vi "VotingClassifier.vi"(8 "error in":errorcluster) -> (0 "error out":errorcluster, 3 "out":refnum<class "VotingClassifier.lvclass">)   [LabVIEW 2020]
doc: "Soft Voting/Majority Rule classifier for unfitted estimators.\n\n Read more in the :ref:`User Guide <voting_classifier>`.\n\n .. versionadded:: 0.17\n\n Parameters\n ----------\n estimators : list of (str, estimator) tuples\n Invoking the ``fit`` method on the ``VotingClassifier`` will fit clones\n of those original estimators that will be stored in the class attribute\n ``self.estimators_``. An estimator can be set to ``'drop'``\n using ``set_params``.\n\n .. versionchanged:: 0.21\n ``'drop'`` is accepted. Using None was deprecated in 0.22 and\n support was removed in 0.24.\n\n voting : {'hard', 'soft'}, default='hard'\n If 'hard', uses predicted class labels for majority rule voting.\n Else if 'soft', predicts the class label based on the argmax of\n the sums of the predicted probabilities, which is recommended for\n an ensemble of well-calibrated classifiers.\n\n weights : array-like of shape (n_classifiers,), default=None\n Sequence of weights (`float` or `int`) to weight the occurrences of\n predicted class labels (`hard` voting) or class probabilities\n before averaging (`soft` voting). Uses uniform weights if `None`.\n\n n_jobs : int, default=None\n The number of jobs to run in parallel for ``fit``.\n ``None`` means 1 unless in a :obj:`joblib.parallel_backend` context.\n ``-1`` means using all processors. See :term:`Glossary <n_jobs>`\n for more details.\n\n .. versionadded:: 0.18\n\n flatten_transform : bool, default=True\n Affects shape of transform output only when voting='soft'\n If voting='soft' and flatten_transform=True, transform method returns\n matrix with shape (n_samples, n_classifiers * n_classes). If\n flatten_transform=False, it returns\n (n_classifiers, n_samples, n_classes).\n\n verbose : bool, default=False\n If True, the time elapsed while fitting will be printed as it\n is completed.\n\n .. versionadded:: 0.23\n\n Attributes\n ----------\n estimators_ : list of classifiers\n The collection of fitted sub-estimators as defined in ``estimators``\n that are not 'drop'.\n\n named_estimators_ : :class:`~sklearn.utils.Bunch`\n Attribute to access any fitted sub-estimators by name.\n\n .. versionadded:: 0.20\n\n classes_ : array-like of shape (n_predictions,)\n The classes labels.\n\n See Also\n --------\n VotingRegressor : Prediction voting regressor.\n\n \nAvailable methods:\nFit Transform\nTransform\nFit\nPredict\nScore\nGet Attributes\nGet Params\nSet Params"
uses:
  VotingClassifier.lvclass
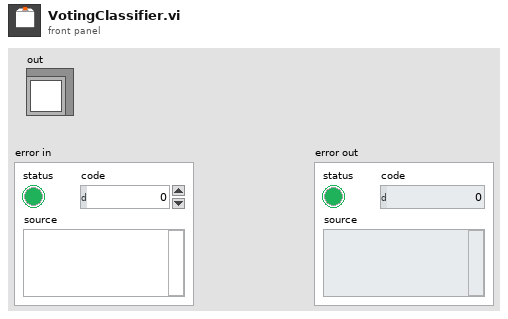
[diagram p1: front panel]
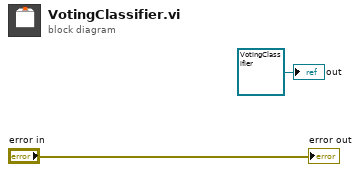
[diagram p0: block diagram]
diagram:
  "out" <- refnum<class "VotingClassifier.lvclass"> refnum ("model")
  "error out" <- "error in"
